vi "Write panel message (SubVI).vi"(3 "Stop BurnIn":refnum<vi>, 4 "rpm":refnum<vi>, 5 "rpm":bool, 6 "PrintTime":bool=TRUE, 7 "Stop":refnum<vi>, 8 "error in (no error)":errorcluster, 9 "Time to wait":dbl, 10 "Strin":string, 11 "String in":refnum<vi>) -> (0 "error out":errorcluster)   [LabVIEW 2017]
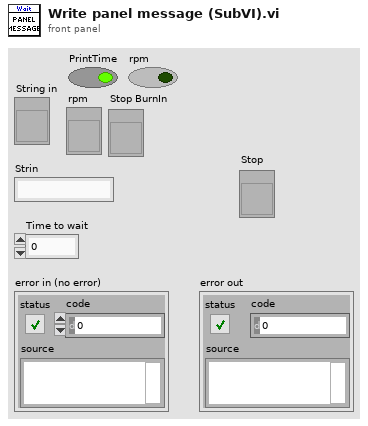
[diagram p1: front panel]
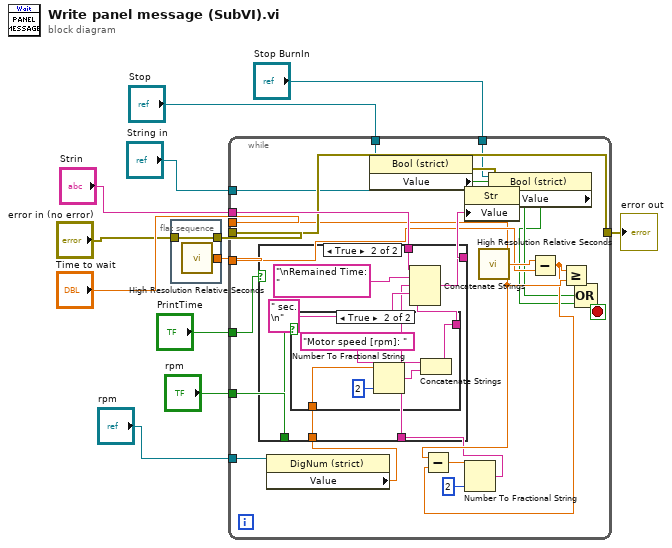
[diagram p0: block diagram]
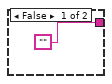
[diagram p3: hidden frame]
diagram:
  n1 = flat-sequence {
    tunnel: [w14] -> w8
    tunnel: "error in (no error)" -> [w14]
    tunnel: [w13] -> w9
    frame #0 {
      n2 = call <vilib>:"High Resolution Relative Seconds.vi"() -> ("relative seconds"=w13:dbl)
    }
  }
  n3 = while {
    tunnel: "Strin" -> [w36]
    tunnel: w8 -> [w31]
    tunnel: w9 -> [w33]
    tunnel: "Time to wait" -> [w27]
    tunnel: [w31] -> w11
    tunnel: "String in" -> [w30]
    tunnel: "Stop" -> [w24]
    tunnel: "PrintTime" -> [w21]
    tunnel: "rpm" -> [w20]
    tunnel: "rpm" -> [w19]
    tunnel: "Stop BurnIn" -> [w15]
    stop <- w23 stop-if-true
    n4 = property class="DigNum (strict)"(reference=w19) -> ("Value"=w18:dbl)  [unwired: 1 in, 2 out]
    n5 = property class="Bool (strict)"(reference=w24) -> (error out=w17:errorcluster, "Value"=w22:bool)  [unwired: 1 in, 1 out]
    n6 = call <vilib>:"High Resolution Relative Seconds.vi"() -> ("relative seconds"=w34:dbl)
    n7 = property class="Bool (strict)"(reference=w15, error in=w17) -> ("Value"=w16:bool)  [unwired: 2 out]
    n8 = Subtract(x=w34, y=w33) -> (x-y=w26:dbl)
    n9 = Subtract(x=w27, y=w26) -> (x-y=w28:dbl)
    n10 = Number To Fractional String(number=w28, precision (6)=i16 2) -> (F-format string=w25:string)  [unwired: 2 in]
    n11 = case shown="True" w21 {
      tunnel: w36 -> [w37 w45]
      tunnel: [w37 w42] -> w35
      tunnel: w25 -> [_ w41]
      tunnel: w20 -> [_ w40]
      tunnel: w18 -> [_ w38]
      frame False {
      }
      frame True {
        n12 = case shown="True" w40 {
          tunnel: ["" w48] -> w39
          tunnel: w38 -> [_ w47]
          frame False {
          }
          frame True {
            n13 = Number To Fractional String(number=w47, precision (6)=i16 2) -> (F-format string=w49:string)  [unwired: 2 in]
            n14 = Concatenate Strings("Motor speed [rpm]: " ("string"), w49) -> (w48:string)
          }
        }
        n15 = Concatenate Strings(w45, "\nRemained Time: " ("string"), w41, " sec.\n" ("string"), w39) -> (w42:string)
      }
    }
    n16 = property class="Str"(reference=w30, "Value"=w35) -> ()  [unwired: 1 in, 2 out]
    n17 = Greater Or Equal?(x=w26, y=w27) -> (x >= y?=w32:bool)
    n18 = Compound Arithmetic op=OR(w32, w22, w16) -> (w23:bool)
  }
  "error out" <- w11
